vi "vcapi.vi"() -> ()   [LabVIEW 2023]
uses:
  RDB/RDB.lvlib
panel:
  out "isComplete":u8
  out "simTime":dbl
  out "simFrame":dbl
  out "error out":errorcluster
  in  "payload":u8[](array[numeric])
  in  "error in (no error)":errorcluster
  in  "path in":path
  out "return type":i32
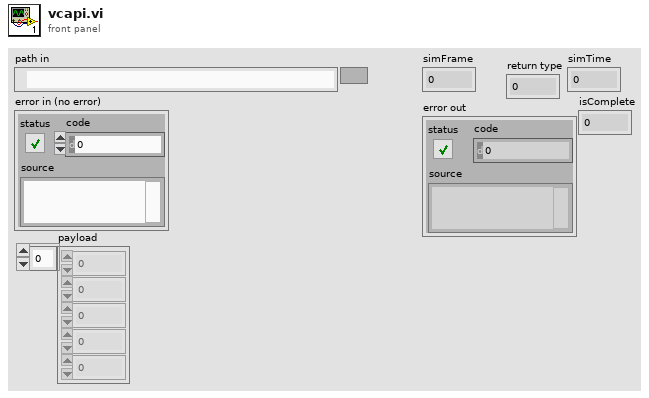
[diagram p1: front panel]
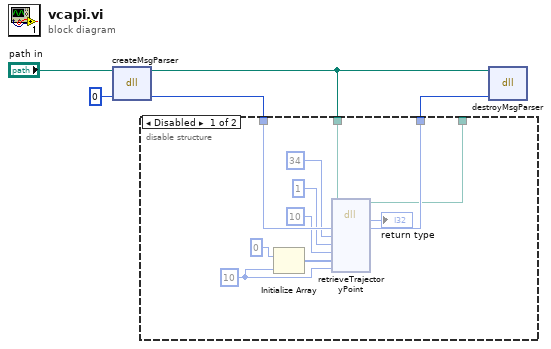
[diagram p0: block diagram]
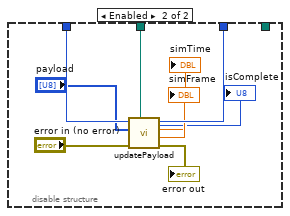
[diagram p2: hidden frame]
diagram:
  n1 = dll-call lib="Z:/VTD/Release/VC.dll" fn="createMsgParser"(path in="path in", "arg1"=u64 0) -> (path out=w1:path, "arg1"=w4:u64)  [unwired: 3 in, 1 out]
  n2 = disable-structure shown="Disabled" {
    disable-tunnel: w4 -> [w16 w24]
    disable-tunnel: [w15 w23] -> w3
    disable-tunnel: w1 -> [w7 w25]
    disable-tunnel: [w6 _] -> _
    frame Disabled {
      w8 = 10 ("dimension size")
      n3 = Initialize Array(u8 0 ("element"), w8) -> (w9:u8[])
      n4 = dll-call lib="Z:/VTD/Release/VC.dll" fn="retrieveTrajectoryPoint"(path in=w7, "handle"=w16, "pkgID"=u16 34, "playerID"=u32 1, "pointIndex"=u16 10, "dataOut"=w9, "dataSz"=w8) -> (path out=w6:path, "return type"=→"return type":i32, "handle"=w15:u64)  [unwired: 7 in, 1 out]
    }
    frame Enabled {
      n5 = call "updatePayload.vi"("path in"=w25, "error in (no error)"="error in (no error)", "payload"="payload", "paeseHandle in"=w24) -> ("error out"=→"error out":errorcluster, "simFrame"=→"simFrame":dbl, "simTime"=→"simTime":dbl, "paeseHandle out"=w23:u64, "isComplete"=→"isComplete":u8)  [unwired: 3 in]
    }
  }
  n6 = dll-call lib="Z:/VTD/Release/VC.dll" fn="destroyMsgParser"(path in=w1, "handle"=w3) -> ()  [unwired: 4 in, 2 out]
